vi "SQLConnect.vi"(4 "Password":string, 5 "error in (no error)":errorcluster, 6 "UserName":string, 7 "ServerName":string, 8 "InputHandle":i32) -> (0 "error out":errorcluster, 3 "OutputHandle":i32)   [LabVIEW 2011]
doc: "Se connecte auprès de la base spécifiée. S'identifie par le nom d'utilisateur et le mot de passe associé"
uses:
  Odbc32.dll
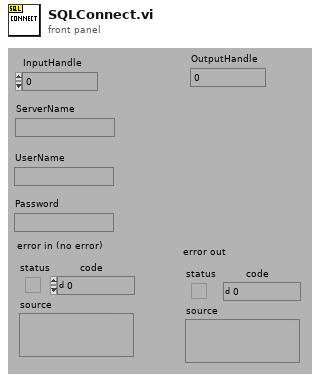
[diagram p1: front panel]
types:
  T1 = enum16{"NOPE", "SQL_HANDLE_ENV", "SQL_HANDLE_DBC", "SQL_HANDLE_STMT", "SQL_HANDLE_DESC"}
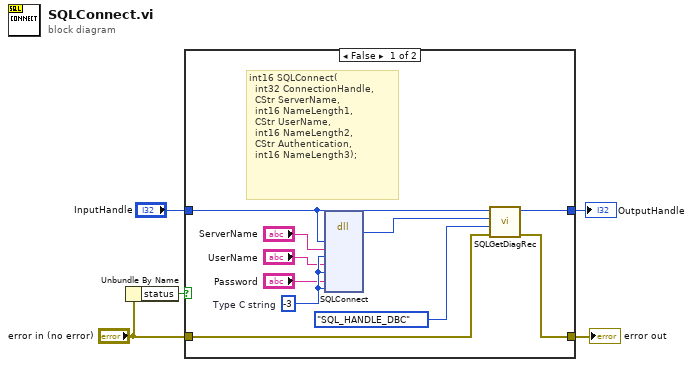
[diagram p0: block diagram]
diagram:
  n1 = Unbundle By Name("error in (no error)") -> ("status"=w4:bool)
  n2 = case shown="False" w4 {
    tunnel: "InputHandle" -> [w11 w17]
    tunnel: "error in (no error)" -> [w9 w16]
    tunnel: [w8 w16] -> w3
    tunnel: [w10 w17] -> w2
    frame False {
      w14 = i16 -3  # Type C string
      # "int16 SQLConnect(\n  int32 ConnectionHandle, \n  CStr ServerName, \n  int16 NameLength1, \n  CStr UserName, \n  int16 NameLength2, \n  CStr Authentication, \n  int16 NameLength3);"
      n3 = dll-call lib="Odbc32.dll" fn="SQLConnect"("ConnectionHandle"=w11, "ServerName"="ServerName", "NameLength1"=w14, "UserName"="UserName", "NameLength2"=w14, "Authentication"="Password", "NameLength3"=w14) -> (w7:i16)  [unwired: 10 in, 2 out]
      n4 = call "SQLGetDiagRec.vi"("error in (no error)"=w9, "HandleType"=T1."SQL_HANDLE_DBC", "Status (SQL_SUCCESS=0)"=w7, "Input Handle"=w11) -> ("error out"=w8:errorcluster, "Output Handle"=w10:i32)  [unwired: 2 out]
    }
    frame True {
    }
  }
  "OutputHandle" <- w2
  "error out" <- w3
